vi "Clear Indicators.vi"(8 "error in":errorcluster, 11 "SwitchMatrix in":refnum<class "SwitchMatrix.lvclass">) -> (0 "error out":errorcluster, 3 "SwitchMatrix out":refnum<class "SwitchMatrix.lvclass">)   [LabVIEW 2019, in "SwitchMatrix.lvlib" / "SwitchMatrix.lvclass"]
uses:
  Library/SwitchMatrix.lvclass
  Library/SwitchMatrix.lvclass/SwitchMatrix.ctl
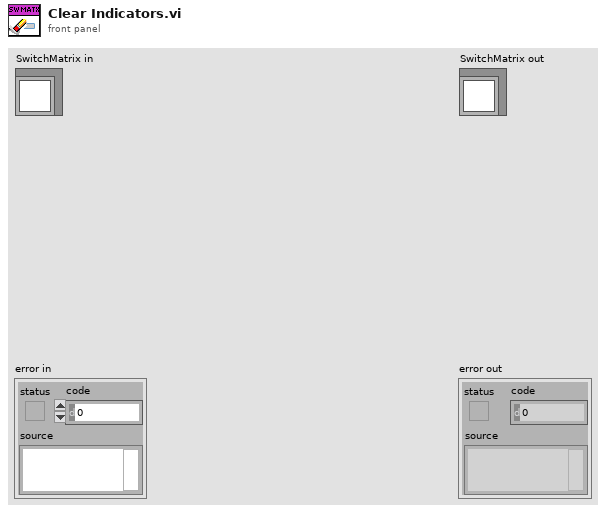
[diagram p1: front panel]
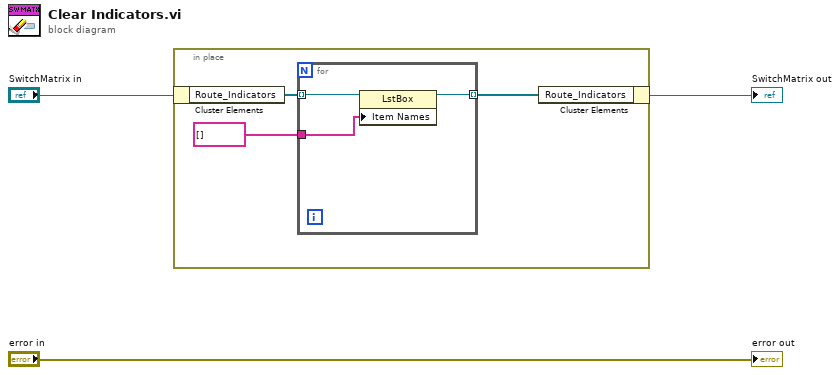
[diagram p0: block diagram]
diagram:
  n1 = in-place {
    n2 = in-place-cluster #1("SwitchMatrix in") -> ("Route_Indicators"=w6:refnum<vi>[])
    n3 = for {
      tunnel: w6 -> [w9] mode=indexing
      tunnel: [w8] -> w5 mode=indexing
      tunnel: string[] [] ("Item Names") -> [w7]
      n4 = property class="LstBox"(reference=w9, "Item Names"=w7) -> (reference out=w8:refnum<vi>)  [unwired: 1 in, 1 out]
    }
    n5 = in-place-cluster #1("Route_Indicators"=w5) -> (→"SwitchMatrix out":refnum<class "SwitchMatrix.lvclass">)
  }
  "error out" <- "error in"
